vi "g_CommandParam.vi"() -> ()   [LabVIEW 2014]
uses:
  c_InstructionEnum.ctl
  c_PlatePosEnum.ctl
panel:
  out "Plate Position":T1=enum."Seperate"
  out "Command":T2=enum."Move Home"
  out "Y Stepsize":dbl
  out "X Stepsize":dbl
  out "Y Steps":dbl
  out "X Steps":dbl
  out "Y":dbl
  out "X":dbl
  # "Absolute Movements"
  # "Increment"
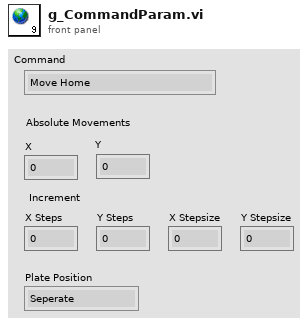
[diagram p1: front panel]
types:
  T1 = typedef "c_PlatePosEnum.ctl" = enum16{"Contact", "Seperate"}
  T2 = typedef "c_InstructionEnum.ctl" = enum16{"Move Absolute", "Increment", "Move Home", "Motion Kill", "Move Plate", "Set Stepsize", "Query Position"}
diagram:
